vi "SVT Set Swept Sine Averaging.vi"(8 "error in (no error)":errorcluster, 9 "integration time":T1={"integration time [s]"=0.015599999576807022, "integration cycles"=5} {"integration cycles" min=2; "integration time [s]" format="%.2p"}, 10 "settling time":T2={"settle time [s]"=0.015599999576807022, "settle cycles"=5} {"settle time [s]" format="%.2p"}, 11 "swept sine task in":T3={"source settings"={"AO task name"="", "source"=[]}, "stimulus settings"={"stimulus task name"="", "stimulus"=[]}, "response(s) settings"={"response task name"="", "response"=[]}, "measurement settings"={"AI sampling frequency"=51200.0, "AO sampling frequency"=1024.0, "AI block size"=1024, "AO block Size"=1024, "block duration [ms]"=1024.0, "number of AI channels"=0, "device propagation delay [samples]"=0.0, "total propagation time [samples]"=0.0, "DUT propagation time [ms]"=0.0}, "linlog"=enum."linear", "repeat"=enum."off", "frequency list"=[1.0], "amplitude list"=[1.0], "settling time"={"settle time"=0.015599999576807022, "settle cycles"=5}, "integration time"={"integration time"=0.015599999576807022, "integration cycles"=5}, "frequencies indices"={"AI freq index"=0, "AO freq index"=5}, "read marks"={"write index"=0, "read index"=0, "freq start index"=0, "freq stop index"=0, "# extracted"=0, "buffer type"=enum."Invalid buffer", "read/write indices"=[], "AO index"=0, "AI index"=0, "settled"=FALSE, "integration done"=FALSE}, "harmonic settings"={"maximum THD harmonic"=5, "harmonic mapping"=[1], "units"={"THD unit"=enum."%", "nth harmonic unit"=enum."%", "SINAD unit"=enum."dB", "THD+N unit"=enum."dB"}}, "auto resolution settings"={"auto max step"=512, "slow threshold db"=6.0, "fast threshold db"=1.0}, "auto level settings"={"auto level enable"=FALSE, "auto level channel"=6, "ideal ref"=1.0, "max level"=10.0, "ref upper deviation db"=3.0, "ref lower deviation db"=-3.0}, "offset"=1.0, "ramping rate"=0.0, "phase"=1.0, "initialize"=FALSE} {"phase" format="%.2f"; "response(s) settings"."response"."channel info"."pregain" format="%.2f"; "response(s) settings"."response"."channel info"."weighting filter" items=["Linear", "A-weighting", "B-weighting", "C-weighting", "ITU-R 468-4", "Dolby", "CCITT", "C-message", "Wb", "Wc", "Wd", "We", "Wf", "Wh", "Wj", "Wk", "Wm", "AES17 20 kHz lowpass", "AES17 40 kHz lowpass", "AES17 20 kHz highpass", "AES17 40 kHz highpass"]; "response(s) settings"."response"."channel info"."dB reference" format="%^.1e"; "response(s) settings"."response"."channel info"."engineering units" items=["custom..."=0, "V"=1, "A"=21, "C"=30, "pC"=31, "s"=32, "-"=29, "Pa"=2, "N"=20, "g"=3, "m/s^2"=4, "m/s"=5, "m"=6, "mm/s"=12, "mm"=13, "micron/s"=14, "micron"=15, "in/s^2"=7, "in/s"=8, "in"=9, "mil/s"=10, "mil"=11, "rad/s^2"=16, "rad/s"=17, "rad"=18, "deg/s^2"=26, "deg/s"=27, "deg"=28, "RPM"=22, "cycle/s^2"=23, "Hz"=24, "cycle"=25, "strain"=19]; "response(s) settings"."response"."channel info"."sensor sensitivity" format="%#_5f"; "stimulus settings"."stimulus"."channel info"."pregain" format="%.2f"; "stimulus settings"."stimulus"."channel info"."weighting filter" items=["Linear", "A-weighting", "B-weighting", "C-weighting", "ITU-R 468-4", "Dolby", "CCITT", "C-message", "Wb", "Wc", "Wd", "We", "Wf", "Wh", "Wj", "Wk", "Wm", "AES17 20 kHz lowpass", "AES17 40 kHz lowpass", "AES17 20 kHz highpass", "AES17 40 kHz highpass"]; "stimulus settings"."stimulus"."channel info"."dB reference" format="%^.1e"; "stimulus settings"."stimulus"."channel info"."engineering units" items=["custom..."=0, "V"=1, "A"=21, "C"=30, "pC"=31, "s"=32, "-"=29, "Pa"=2, "N"=20, "g"=3, "m/s^2"=4, "m/s"=5, "m"=6, "mm/s"=12, "mm"=13, "micron/s"=14, "micron"=15, "in/s^2"=7, "in/s"=8, "in"=9, "mil/s"=10, "mil"=11, "rad/s^2"=16, "rad/s"=17, "rad"=18, "deg/s^2"=26, "deg/s"=27, "deg"=28, "RPM"=22, "cycle/s^2"=23, "Hz"=24, "cycle"=25, "strain"=19]; "stimulus settings"."stimulus"."channel info"."sensor sensitivity" format="%#_5f"; "ramping rate" format="%.4f"; "offset" format="%.2f"; "auto level settings"."ref lower deviation db" format="%.4f"; "auto level settings"."ref upper deviation db" format="%.4f"; "auto level settings"."max level" format="%.4f"; "auto level settings"."ideal ref" format="%.4f"; "auto resolution settings"."fast threshold db" format="%.4f"; "auto resolution settings"."slow threshold db" format="%.4f"; "harmonic settings"."maximum THD harmonic" max=10 step=1; "integration time"."integration time" format="%.2p"; "settling time"."settle time" format="%.2p"; "amplitude list" format="%.2f"; "frequency list" format="%.2f"; "measurement settings"."DUT propagation time [ms]" format="%.2f"; "measurement settings"."AO sampling frequency" format="%.2f"; "measurement settings"."AI sampling frequency" format="%.2f"}) -> (0 "error out":errorcluster, 3 "swept sine task out":T3={"source settings"={"AO task name"="", "source"=[]}, "stimulus settings"={"stimulus task name"="", "stimulus"=[]}, "response(s) settings"={"response task name"="", "response"=[]}, "measurement settings"={"AI sampling frequency"=51200.0, "AO sampling frequency"=1024.0, "AI block size"=1024, "AO block Size"=1024, "block duration [ms]"=1024.0, "number of AI channels"=0, "device propagation delay [samples]"=0.0, "total propagation time [samples]"=0.0, "DUT propagation time [ms]"=0.0}, "linlog"=enum."linear", "repeat"=enum."off", "frequency list"=[1.0], "amplitude list"=[1.0], "settling time"={"settle time"=0.015599999576807022, "settle cycles"=5}, "integration time"={"integration time"=0.015599999576807022, "integration cycles"=5}, "frequencies indices"={"AI freq index"=0, "AO freq index"=5}, "read marks"={"write index"=0, "read index"=0, "freq start index"=0, "freq stop index"=0, "# extracted"=0, "buffer type"=enum."Invalid buffer", "read/write indices"=[], "AO index"=0, "AI index"=0, "settled"=FALSE, "integration done"=FALSE}, "harmonic settings"={"maximum THD harmonic"=5, "harmonic mapping"=[1], "units"={"THD unit"=enum."%", "nth harmonic unit"=enum."%", "SINAD unit"=enum."dB", "THD+N unit"=enum."dB"}}, "auto resolution settings"={"auto max step"=512, "slow threshold db"=6.0, "fast threshold db"=1.0}, "auto level settings"={"auto level enable"=FALSE, "auto level channel"=6, "ideal ref"=1.0, "max level"=10.0, "ref upper deviation db"=3.0, "ref lower deviation db"=-3.0}, "offset"=1.0, "ramping rate"=0.0, "phase"=1.0, "initialize"=FALSE} {"phase" format="%.2f"; "response(s) settings"."response"."channel info"."pregain" format="%.2f"; "response(s) settings"."response"."channel info"."weighting filter" items=["Linear", "A-weighting", "B-weighting", "C-weighting", "ITU-R 468-4", "Dolby", "CCITT", "C-message", "Wb", "Wc", "Wd", "We", "Wf", "Wh", "Wj", "Wk", "Wm", "AES17 20 kHz lowpass", "AES17 40 kHz lowpass", "AES17 20 kHz highpass", "AES17 40 kHz highpass"]; "response(s) settings"."response"."channel info"."dB reference" format="%^.1e"; "response(s) settings"."response"."channel info"."engineering units" items=["custom..."=0, "V"=1, "A"=21, "C"=30, "pC"=31, "s"=32, "-"=29, "Pa"=2, "N"=20, "g"=3, "m/s^2"=4, "m/s"=5, "m"=6, "mm/s"=12, "mm"=13, "micron/s"=14, "micron"=15, "in/s^2"=7, "in/s"=8, "in"=9, "mil/s"=10, "mil"=11, "rad/s^2"=16, "rad/s"=17, "rad"=18, "deg/s^2"=26, "deg/s"=27, "deg"=28, "RPM"=22, "cycle/s^2"=23, "Hz"=24, "cycle"=25, "strain"=19]; "response(s) settings"."response"."channel info"."sensor sensitivity" format="%#_5f"; "stimulus settings"."stimulus"."channel info"."pregain" format="%.2f"; "stimulus settings"."stimulus"."channel info"."weighting filter" items=["Linear", "A-weighting", "B-weighting", "C-weighting", "ITU-R 468-4", "Dolby", "CCITT", "C-message", "Wb", "Wc", "Wd", "We", "Wf", "Wh", "Wj", "Wk", "Wm", "AES17 20 kHz lowpass", "AES17 40 kHz lowpass", "AES17 20 kHz highpass", "AES17 40 kHz highpass"]; "stimulus settings"."stimulus"."channel info"."dB reference" format="%^.1e"; "stimulus settings"."stimulus"."channel info"."engineering units" items=["custom..."=0, "V"=1, "A"=21, "C"=30, "pC"=31, "s"=32, "-"=29, "Pa"=2, "N"=20, "g"=3, "m/s^2"=4, "m/s"=5, "m"=6, "mm/s"=12, "mm"=13, "micron/s"=14, "micron"=15, "in/s^2"=7, "in/s"=8, "in"=9, "mil/s"=10, "mil"=11, "rad/s^2"=16, "rad/s"=17, "rad"=18, "deg/s^2"=26, "deg/s"=27, "deg"=28, "RPM"=22, "cycle/s^2"=23, "Hz"=24, "cycle"=25, "strain"=19]; "stimulus settings"."stimulus"."channel info"."sensor sensitivity" format="%#_5f"; "ramping rate" format="%.4f"; "offset" format="%.2f"; "auto level settings"."ref lower deviation db" format="%.4f"; "auto level settings"."ref upper deviation db" format="%.4f"; "auto level settings"."max level" format="%.4f"; "auto level settings"."ideal ref" format="%.4f"; "auto resolution settings"."fast threshold db" format="%.4f"; "auto resolution settings"."slow threshold db" format="%.4f"; "harmonic settings"."maximum THD harmonic" max=10 step=1; "integration time"."integration time" format="%.2p"; "settling time"."settle time" format="%.2p"; "amplitude list" format="%.2f"; "frequency list" format="%.2f"; "measurement settings"."DUT propagation time [ms]" format="%.2f"; "measurement settings"."AO sampling frequency" format="%.2f"; "measurement settings"."AI sampling frequency" format="%.2f"})   [LabVIEW 2017, in "SoundVib_SweptSine.lvlib"]
doc: "Configures the sine-sweep settling time and integration time settings."
uses:
  <vilib>/addons/Sound and Vibration/svt_Swept Sine/SoundVib_SweptSine.lvlib
  <vilib>/addons/Sound and Vibration/svt_Swept Sine/subVIs/sv_Swept Sine Task.ctl
  <vilib>/addons/_NISVFA/_Shared subVIs/Controls/svc_Channel Info.ctl
  <vilib>/addons/_NISVFA/_Shared subVIs/Controls/svc_Engineering Units Text Ring.ctl
  <vilib>/addons/_NISVFA/_Shared subVIs/Controls/svc_Weighting Filter Text Ring.ctl
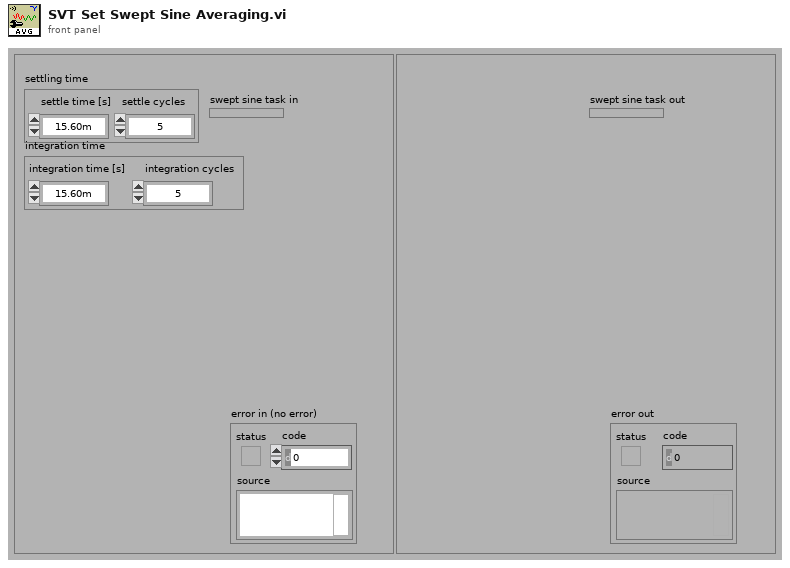
[diagram p1: front panel]
types:
  T1 = cluster{"integration time [s]":dbl, "integration cycles":i32}
  T2 = cluster{"settle time [s]":dbl, "settle cycles":i32}
  T3 = typedef "SoundVib_SweptSine.lvlib/sv_Swept Sine Task.ctl" = cluster{"source settings":cluster{"AO task name":refnum<k21>, "source":cluster{"AO physical channel":tag}[]}, "stimulus settings":cluster{"stimulus task name":refnum<k21>, "stimulus":cluster{"stimulus physical channel":tag, "channel info":T4}[]}, "response(s) settings":cluster{"response task name":refnum<k21>, "response":cluster{"response physical channel":tag, "channel info":T4}[]}, "measurement settings":cluster{"AI sampling frequency":dbl, "AO sampling frequency":dbl, "AI block size":i32, "AO block Size":i32, "block duration [ms]":dbl, "number of AI channels":i32, "device propagation delay [samples]":dbl, "total propagation time [samples]":dbl, "DUT propagation time [ms]":dbl}, "linlog":enum16{"linear", "log"}, "repeat":enum16{"off", "on"}, "frequency list":dbl[], "amplitude list":dbl[], "settling time":cluster{"settle time":dbl, "settle cycles":i32}, "integration time":cluster{"integration time":dbl, "integration cycles":i32}, "frequencies indices":cluster{"AI freq index":i32, "AO freq index":i32}, "read marks":cluster{"write index":u32, "read index":u32, "freq start index":u32, "freq stop index":u32, "# extracted":u32, "buffer type":enum16{"Invalid buffer", "Intermediate buffer", "Final buffer"}, "read/write indices":cluster{"settle time index":u32, "integration time index":u32}[], "AO index":i32, "AI index":i32, "settled":bool, "integration done":bool}, "harmonic settings":cluster{"maximum THD harmonic":u32, "harmonic mapping":u32[], "units":cluster{"THD unit":enum16{"dB", "%"}, "nth harmonic unit":enum16{"dB", "%"}, "SINAD unit":enum16{"dB", "%"}, "THD+N unit":enum16{"dB", "%"}}}, "auto resolution settings":cluster{"auto max step":i32, "slow threshold db":dbl, "fast threshold db":dbl}, "auto level settings":cluster{"auto level enable":bool, "auto level channel":u8, "ideal ref":sgl, "max level":sgl, "ref upper deviation db":sgl, "ref lower deviation db":sgl}, "offset":dbl, "ramping rate":dbl, "phase":dbl, "initialize":bool}
  T4 = typedef "svc_Channel Info.ctl" = cluster{"sensor sensitivity":dbl, "engineering units":T5, "dB reference":dbl, "custom label":string, "weighting filter":T6, "pregain":dbl}
  T5 = typedef "svc_Engineering Units Text Ring.ctl" = u16
  T6 = typedef "svc_Weighting Filter Text Ring.ctl" = u16
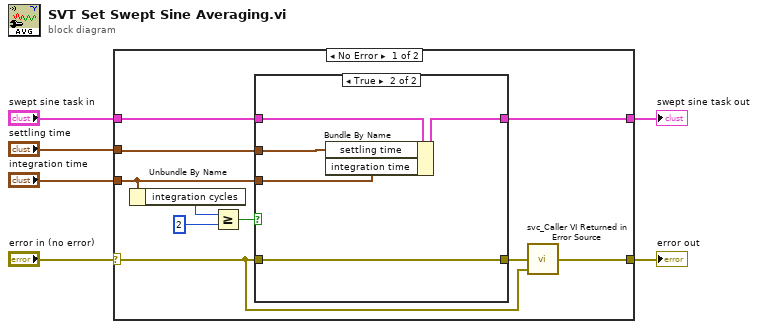
[diagram p0: block diagram]
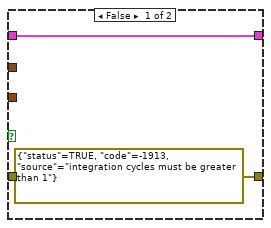
[diagram p2: hidden frame]
diagram:
  n1 = case shown="No Error" "error in (no error)" {
    selector: "error in (no error)" -> [w7 w25]
    tunnel: "settling time" -> [w11 _]
    tunnel: "integration time" -> [w10 _]
    tunnel: "swept sine task in" -> [w13 w24]
    tunnel: [w12 w24] -> w3
    tunnel: [w8 w25] -> w1
    frame No Error {
      n2 = Unbundle By Name(w10) -> ("integration cycles"=w16:i32)
      n3 = Greater Or Equal?(x=w16, y=2) -> (x >= y?=w15:bool)
      n4 = case shown="True" w15 {
        tunnel: w7 -> [_ w23]
        tunnel: [errorcluster {"status"=TRUE, "code"=-1913, "source"="integration cycles must be greater than 1"} ("error IO") w23] -> w9
        tunnel: w13 -> [w18 w20]
        tunnel: [w18 w19] -> w12
        tunnel: w11 -> [_ w22]
        tunnel: w10 -> [_ w21]
        frame False {
        }
        frame True {
          n5 = Bundle By Name(cluster=w20, "settling time"=w22, "integration time"=w21) -> (w19:T3)
        }
      }
      n6 = call <vilib>:"svc_Caller VI Returned in Error Source.vi"("warning input to caller"=w7, "error in (no error)"=w9) -> ("error out"=w8:errorcluster)  [unwired: 3 in]
    }
    frame Error {
    }
  }
  "error out" <- w1
  "swept sine task out" <- w3
